vi "波形图表接受的数据类型.vi"() -> ()   [LabVIEW 2010]
uses:
  Instance           1 27Saved   chart接受的数据类型 .vi
  <vilib>/Analysis/NI_AALBase.lvlib
  <vilib>/measure/NI_MABase.lvlib
panel:
  out "波形图表":dynamicdata(graph)
  out "波形图表":waveform(dbl)(graph)
  out "波形图表":waveform(dbl)[](graph)
  out "波形图表":dbl[](graph)
  out "波形图表":cluster{"number: 0 to 1":dbl, dbl}[](graph)
  out "波形图表":dbl[][](graph)
  out "波形图表":dbl(graph)
  out "波形图表":cluster{"number: 0 to 1":dbl, dbl}(graph)
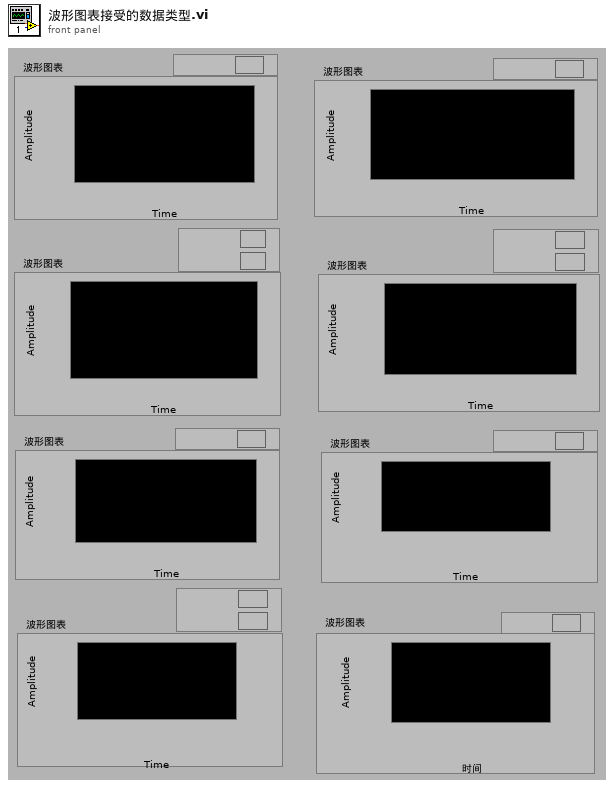
[diagram p1: front panel]
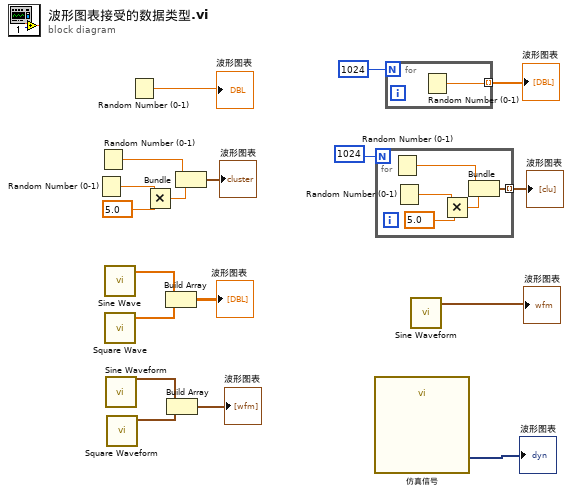
[diagram p0: block diagram]
diagram:
  n1 = Random Number (0-1)() -> (number: 0 to 1=w18:dbl)
  n2 = Random Number (0-1)() -> (number: 0 to 1=w15:dbl)
  n3 = call <vilib>:"Sine Wave.vi"() -> ("sine wave"=w10:dbl[])  [unwired: 5 in, 2 out]
  n4 = call <vilib>:"Square Wave.vi"() -> ("square wave"=w11:dbl[])  [unwired: 6 in, 2 out]
  n5 = call <vilib>:"Sine Waveform.vi"() -> ("signal out"=w4:waveform(dbl))  [unwired: 10 in, 1 out]
  n6 = call <vilib>:"Square Waveform.vi"() -> ("signal out"=w3:waveform(dbl))  [unwired: 10 in, 1 out]
  n7 = Random Number (0-1)() -> (number: 0 to 1=→"波形图表":dbl)
  n8 = Multiply(x=w18, y=5.0) -> (x*y=w16:dbl)
  n9 = Build Array(w10, w11) -> (→"波形图表":dbl[][])
  n10 = Build Array(w4, w3) -> (→"波形图表":waveform(dbl)[])
  n11 = Bundle("number: 0 to 1"=w15, w16) -> (→"波形图表":cluster{"number: 0 to 1":dbl, dbl})  [unwired: 1 in]
  n12 = call "仿真信号"() -> ("正弦"=→"波形图表":dynamicdata)  [unwired: 14 in, 1 out]
  n13 = for {
    N: 1024 -> [_]
    tunnel: [w19] -> w8 mode=indexing
    n14 = Random Number (0-1)() -> (number: 0 to 1=w20:dbl)
    n15 = Random Number (0-1)() -> (number: 0 to 1=w23:dbl)
    n16 = Multiply(x=w23, y=5.0) -> (x*y=w21:dbl)
    n17 = Bundle("number: 0 to 1"=w20, w21) -> (w19:cluster{"number: 0 to 1":dbl, dbl})  [unwired: 1 in]
  }
  "波形图表" <- w8
  n18 = for {
    N: 1024 -> [_]
    tunnel: [w24] -> w7 mode=indexing
    n19 = Random Number (0-1)() -> (number: 0 to 1=w24:dbl)
  }
  "波形图表" <- w7
  n20 = call <vilib>:"Sine Waveform.vi"() -> ("signal out"=→"波形图表":waveform(dbl))  [unwired: 10 in, 1 out]
